vi "calibrateValue.vi"(8 "error in (no error)":errorcluster, 10 "value":string, 11 "Channel in":refnum<class "Channel.lvclass">) -> (0 "error out":errorcluster, 2 "calibratedValue":dbl, 3 "Channel out":refnum<class "Channel.lvclass">)   [LabVIEW 2009, in "Tools.lvlib" / "DatabaseHelpers.lvlib" / "Channel.lvclass"]
uses:
  Channel.lvclass
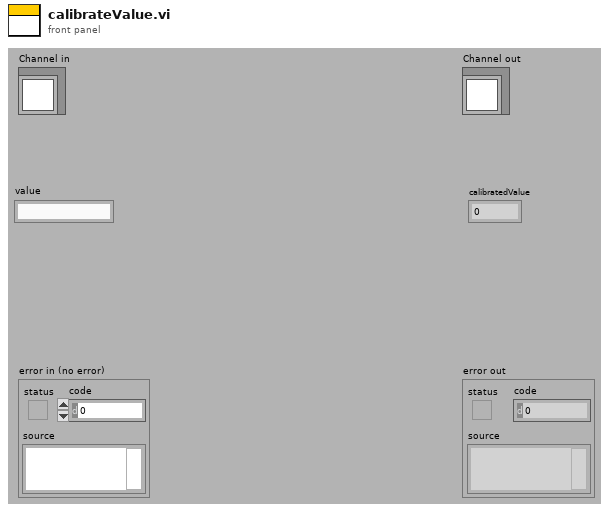
[diagram p1: front panel]
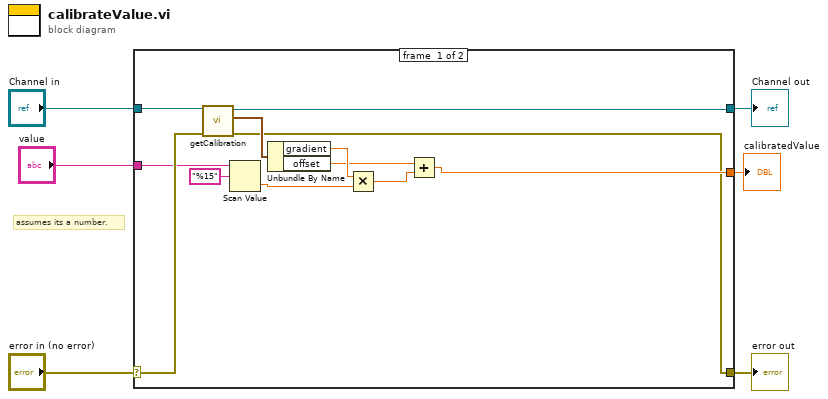
[diagram p0: block diagram]
diagram:
  # "assumes its a number."
  n1 = case shown="No Error" "error in (no error)" {
    selector: "error in (no error)" -> [w16 w20]
    tunnel: [w7 w20] -> w5
    tunnel: [w17 w19] -> w4
    tunnel: "Channel in" -> [w18 w19]
    tunnel: "value" -> [w15 _]
    tunnel: [w8 _] -> w1
    frame #0 {
      n2 = call "getCalibration.vi"("error in (no error)"=w16, "Channel.lvclass in"=w18) -> ("error out"=w7:errorcluster, "calibration"=w13:cluster{"gradient":dbl, "offset":dbl}, "Channel.lvclass out"=w17:refnum<class "Channel.lvclass">)  [unwired: 7 in]
      n3 = Scan Value(string=w15, format string="%15") -> (value=w11:dbl)  [unwired: 1 in, 1 out]
      n4 = Unbundle By Name(w13) -> ("gradient"=w12:dbl, "offset"=w9:dbl)
      n5 = Multiply(x=w12, y=w11) -> (x*y=w10:dbl)
      n6 = Add(x=w9, y=w10) -> (x+y=w8:dbl)
    }
    frame #1 {
    }
  }
  "error out" <- w5
  "Channel out" <- w4
  "calibratedValue" <- w1
